vi "RAW Event.vi"(0 "connection info":T1, 5 "State Variables":T3, 7 "Address Lookup Table":variant, 9 "Identifier":u32 format="%08x", 11 "Data":u8[](array[numeric])=[0, 0, 0, 0, 0, 0, 0, 0], 12 "Error Q":refnum<queue>, 13 "VI Ref":refnum<vi>) -> (4 "connection info":T1, 8 "Address Lookup Table Out":variant)   [LabVIEW 2023, in "J1939 Workspace Shared.lvlib"]
uses:
  J1939 Workspace Shared.lvlib
  Types/Private Data.ctl
  Addon/Addon Shared/Types/Error Cluster.ctl
  Addon/Addon Shared/Types/Error Types.ctl
  <vilib>/NI/STM/TCP/TCP Connection Info.ctl
  <vilib>/NI/STM/SubVIs/MetaDataElement.ctl
  Addon/Support Libraries/J1939 Utilities/SubVIs/Convert CAN Arb ID to J1939 ID.vi
  Addon/Addon Shared/J1939 Addon Shared.lvlib
  Addon/Support Libraries/J1939 Utilities/J1939 Utilities.lvlib
  <vilib>/NI/STM/NI STM.lvlib
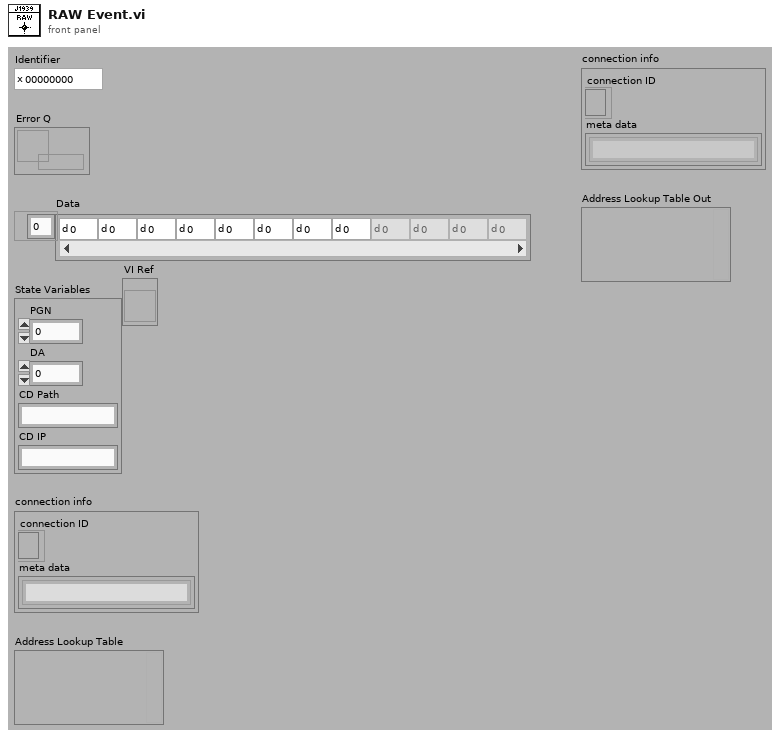
[diagram p1: front panel]
types:
  T1 = typedef "NI STM.lvlib/TCP Connection Info.ctl" = cluster{"connection ID":refnum<k5>, "meta data":T2[]}
  T2 = typedef "NI STM.lvlib/MetaDataElement.ctl" = string
  T3 = typedef "J1939 Workspace Shared.lvlib/Private Data.ctl" = cluster{"PGN":u32, "DA":u8, "CD Path":string, "CD IP":string}
  T4 = typedef "J1939 Addon Shared.lvlib/Error Types.ctl" = enum16{"Request", "RAW Generation", "Clear Active DTCs", "Clear Previous DTCs", "Addresses", "TLAs", "Get Active DTCs", "Get Previous DTCs", "TCP Connection"}
  T5 = typedef "J1939 Addon Shared.lvlib/Error Cluster.ctl" = cluster{"error out":errorcluster, "Enum":T4, "Address":u8, "Timestamp":timestamp}
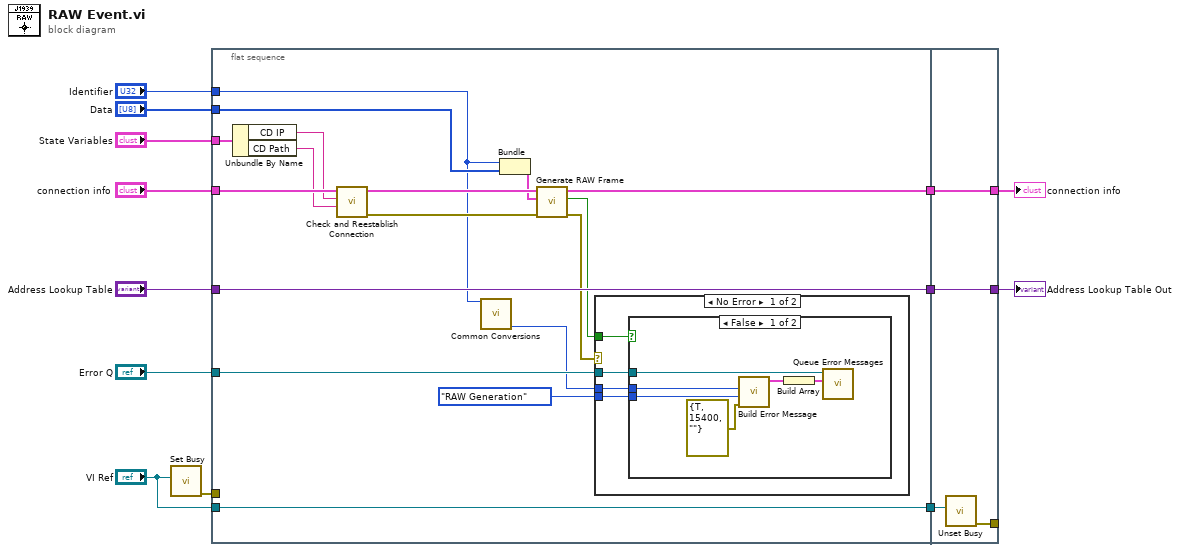
[diagram p0: block diagram]
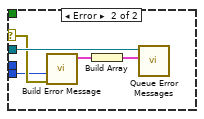
[diagram p3: hidden frame]
diagram:
  n1 = call <vilib>:"Set Busy.vi"("VI reference (current VI)"="VI Ref") -> ("error out"=w7:errorcluster)  [unwired: 9 in, 1 out]
  n2 = flat-sequence {
    tunnel: "connection info" -> [w30]
    tunnel: w7 -> [_]
    tunnel: [w18] -> w13
    tunnel: [w26] -> w12
    tunnel: "Address Lookup Table" -> [w26]
    tunnel: "Error Q" -> [w25]
    tunnel: "State Variables" -> [w22]
    tunnel: "VI Ref" -> [w19]
    tunnel: [w19] -> w3
    tunnel: "Identifier" -> [w15]
    tunnel: "Data" -> [w17]
    tunnel: [w49] -> w6
    tunnel: w13 -> [w49]
    tunnel: [w48] -> _
    tunnel: [w47] -> w8
    tunnel: w12 -> [w47]
    tunnel: w3 -> [w46]
    frame #0 {
      n3 = Unbundle By Name(w22) -> ("CD IP"=w21:string, "CD Path"=w20:string)
      n4 = call "Check and Reestablish Connection.vi"("CD Path"=w20, "IP Address"=w21, "connection info"=w30) -> ("error out"=w29:errorcluster, "connection info"=w28:T1)  [unwired: 7 in]
      n5 = call-poly "Common Conversions.vi"("Arb ID"=w15) -> ("Source Address"=w14:u8)  [unwired: 11 in, 3 out]
      n6 = Bundle("Identifier"=w15, "Data"=w17) -> (w27:cluster{"Identifier":u32, "Data":u8[]})  [unwired: 1 in]
      n7 = call "Generate RAW Frame.vi"("error in (no error)"=w29, "Data to Send"=w27, "connection info"=w28) -> ("error out"=w24:errorcluster, "Sent?"=w16:bool, "connection info"=w18:T1)  [unwired: 6 in]
      n8 = case shown="No Error" w24 {
        selector: w24 -> [_ w44]
        tunnel: w25 -> [w32 w45]
        tunnel: Error_Types."RAW Generation" ("Enum") -> [w33 w41]
        tunnel: w16 -> [w34 _]
        tunnel: w14 -> [w31 _]
        frame No Error {
          n9 = case shown="False" w34 {
            tunnel: w33 -> [w37 _]
            tunnel: w32 -> [w36 _]
            tunnel: w31 -> [w35 _]
            frame False {
              n10 = call "Build Error Message.vi"("error IO"=errorcluster {"status"=TRUE, "code"=15400, "source"=""}, "Enum"=w37, "Address"=w35) -> ("Error Cluster"=w40:T5)  [unwired: 8 in]
              n11 = Build Array(w40) -> (w39:T5[])
              n12 = call "Queue Error Messages.vi"("Error Array"=w39, "queue out"=w36) -> ()  [unwired: 9 in, 1 out]
            }
            frame True {
            }
          }
        }
        frame Error {
          n13 = call "Build Error Message.vi"("error IO"=w44, "Enum"=w41) -> ("Error Cluster"=w43:T5)  [unwired: 9 in]
          n14 = Build Array(w43) -> (w42:T5[])
          n15 = call "Queue Error Messages.vi"("Error Array"=w42, "queue out"=w45) -> ()  [unwired: 9 in, 1 out]
        }
      }
    }
    frame #1 {
      n16 = call <vilib>:"Unset Busy.vi"("VI reference (current VI)"=w46) -> ("error out"=w48:errorcluster)  [unwired: 10 in]
    }
  }
  "Address Lookup Table Out" <- w8
  "connection info" <- w6
